vi "Add Subsystems to Tree.vi"(8 "error in (no error)":errorcluster, 9 "Subsystem I/O Attributes":T1[](array[typedef]), 10 "Subsystems":T4[](array[typedef]), 11 "Tree Control":refnum<vi>) -> (0 "error out":errorcluster, 3 "dup Tree Control":refnum<vi>)   [LabVIEW 2024]
doc: "Adds subsystems to the tree control."
uses:
  Controls/Server/Subsystem Configuration.ctl
  Controls/Server/Subsystem IO Attributes.ctl
  Controls/Server/Subsystem IO Logging Attributes.ctl
  Controls/Server/Subsystem IO Alarm Attributes.ctl
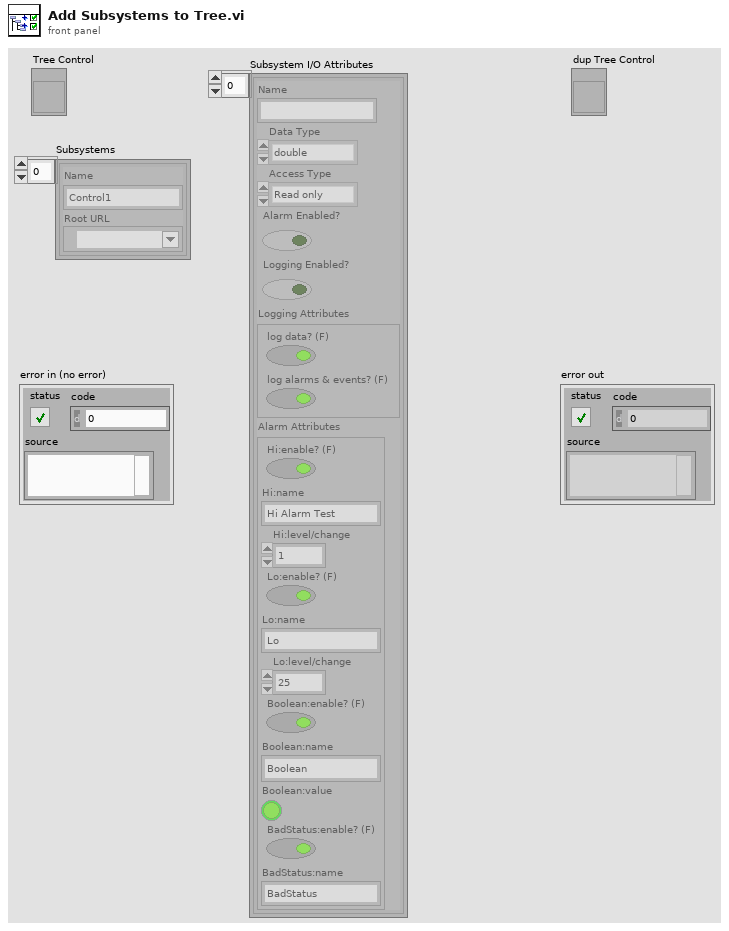
[diagram p1: front panel]
types:
  T1 = typedef "Subsystem IO Attributes.ctl" = cluster{"Name":string, "Data Type":enum32{"u32BitField", "bool", "double", "string", "int8", "uint8", "int16", "uint16", "int32", "uint32", "int64", "uint64", "single", "double waveform", "int16 waveform", "array of boolean", "array of int8", "array of uint8", "array of int16", "array of uint16", "array of int32", "array of uint32", "array of int64", "array of uint64", "array of single", "array of double", "array of double waveform", "array of int16 waveform", "array of string", "variant", "timestamp", "fixed point", "custom"}, "Access Type":enum32{"Read only", "Write only", "Read/write"}, "Alarm Enabled?":bool, "Logging Enabled?":bool, "Logging Attributes":T2, "Alarm Attributes":T3}
  T2 = typedef "Subsystem IO Logging Attributes.ctl" = cluster{"log data? (F)":bool, "log alarms & events? (F)":bool}
  T3 = typedef "Subsystem IO Alarm Attributes.ctl" = cluster{"Hi:enable? (F)":bool, "Hi:name":string, "Hi:level/change":dbl, "Lo:enable? (F)":bool, "Lo:name":string, "Lo:level/change":dbl, "Boolean:enable? (F)":bool, "Boolean:name":string, "Boolean:value":bool, "BadStatus:enable? (F)":bool, "BadStatus:name":string}
  T4 = typedef "Subsystem Configuration.ctl" = cluster{"Name":string, "Root URL":refnum<k21>}
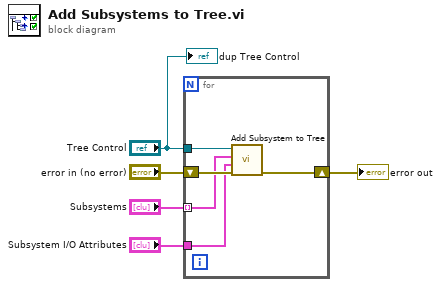
[diagram p0: block diagram]
diagram:
  n1 = for {
    tunnel: "Subsystems" -> [w8] mode=indexing
    shift-right: [w9] -> w2
    shift-left: "error in (no error)" -> [w10]
    tunnel: "Subsystem I/O Attributes" -> [w7]
    tunnel: "Tree Control" -> [w6]
    n2 = call "Add Subsystem to Tree.vi"("error in (no error)"=w10, "Subsystem I/O Attributes"=w7, "Subsystem"=w8, "Tree Control"=w6) -> ("error out"=w9:errorcluster)  [unwired: 6 in, 1 out]
  }
  "error out" <- w2
  "dup Tree Control" <- "Tree Control"
